vi "table-constructor.vi"(7 "table.ref in":refnum<vi>, 8 "error in (no error)":errorcluster, 11 "CANtable in":refnum<class "bAPPdata.lvclass">) -> (0 "error out":errorcluster, 3 "CANtable out":refnum<class "bAPPdata.lvclass">)   [LabVIEW 2015, in "bAPPdata.lvclass"]
uses:
  bAPPdata.lvclass
  CAN_table.ctl
  table-data.ctl
  table-contents.ctl
  subs/frame.type.ctl
  <vilib>/xnet/xnet.llb/XNET Frame CAN.ctl
  <vilib>/xnet/xnet.llb/XNET Frame Type CAN.ctl
  nMsgData.ctl
  bAPPdata.lvclass/bAPPdata.ctl
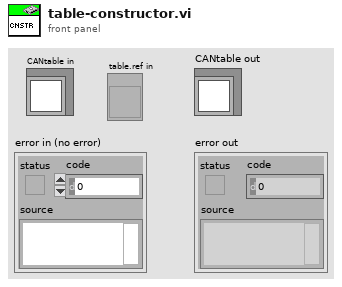
[diagram p1: front panel]
types:
  T1 = typedef "bAPPdata.lvclass/table-data.ctl" = T2[]
  T2 = typedef "bAPPdata.lvclass/table-contents.ctl" = cluster{"id":u32, "tag":string, "frame.type":T3, "last.frame":T4, "tMsgData":T6, "child.tags":string[], "bit-payload":bool[]}
  T3 = typedef "frame.type.ctl" = enum16{"FRAME NOT DEFINED", "DUT OUTPUT FRAME", "DUT INPUT FRAME"}
  T4 = typedef "XNET Frame CAN.ctl" = cluster{"timestamp":timestamp, "payload":u8[], "identifier":u32, "type":T5, "extended?":bool, "echo?":bool}
  T5 = typedef "XNET Frame Type CAN.ctl" = u8
  T6 = typedef "nMsgData.ctl" = cluster{"dwID":u32, "count":u32, "dwCycleTime":dbl, "dwTime":dbl, "new msg":bool}
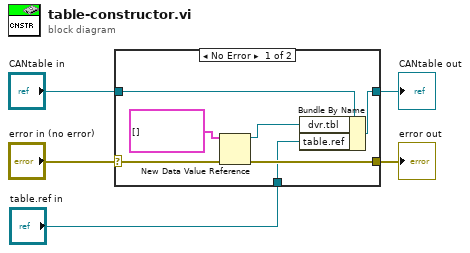
[diagram p0: block diagram]
diagram:
  n1 = case shown="No Error" "error in (no error)" {
    selector: "error in (no error)" -> [w11 w14]
    tunnel: [w10 w14] -> w4
    tunnel: [w8 w13] -> w2
    tunnel: "CANtable in" -> [w12 w13]
    tunnel: "table.ref in" -> [w6 _]
    frame No Error {
      n2 = New Data Value Reference(data value=T1 [] ("tbl.dta"), error in=w11) -> (data value reference=w7:refnum<data-value>, error out=w10:errorcluster)
      n3 = Bundle By Name(cluster=w12, "dvr.tbl"=w7, "table.ref"=w6) -> (w8:refnum<class "bAPPdata.lvclass">)
    }
    frame Error {
    }
  }
  "error out" <- w4
  "CANtable out" <- w2
